vi "2_4.vi"() -> ()   [LabVIEW 2010]
panel:
  out "XY Graph":cluster{dbl[], dbl[]}(graph)
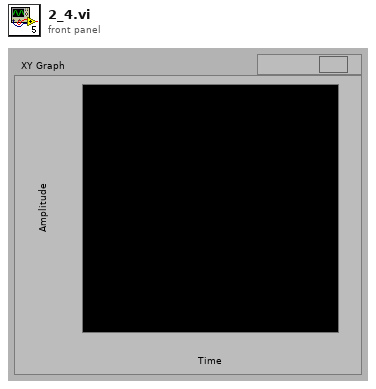
[diagram p1: front panel]
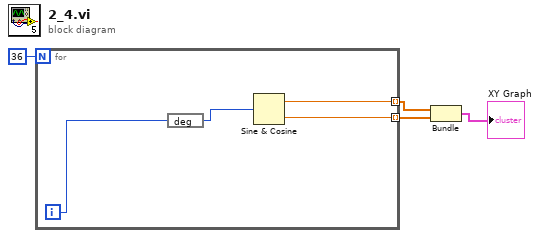
[diagram p0: block diagram]
diagram:
  n1 = for {
    N: 36 -> [_]
    tunnel: [w8] -> w3 mode=indexing
    tunnel: [w7] -> w2 mode=indexing
    i -> [w5]
    n2 = expression code="deg"(w5) -> (w6:i32)
    n3 = Sine & Cosine(0:w6) -> (1:w8:dbl, 2:w7:dbl)
  }
  n4 = Bundle(w3, w2) -> (→"XY Graph":cluster{dbl[], dbl[]})  [unwired: 1 in]
